vi "VCO-FM-1.vi"() -> ()   [LabVIEW 2012]
uses:
  <vilib>/Platform/TimedLoop/XDataNode/timing_clust.ctl
  <vilib>/Platform/TimedLoop/XDataNode/nitl_modes.ctl
  <vilib>/Platform/TimedLoop/XDataNode/wakeup.ctl
  <vilib>/rvi/FXPMathLib/basic elements/FxpIntAccumulator/subVIs/nifxpmath_IntAccumulator_SimConfig.ctl
  <vilib>/rvi/FXPMathLib/FxpSinAndCos/subVIs/nifxpmath_SinAndCos_SimConfig.ctl
  <vilib>/rvi/Emulation/niFpgaSctlEmulationRegisterWithScheduler.vi
  <vilib>/rvi/FXPMathLib/basic elements/FxpIntAccumulator/simVIs/DllFxpIntAccumulator_sub.vi
  <vilib>/rvi/Emulation/niFpgaSctlEmulationScheduler.vi
  <vilib>/rvi/interface/RandomDataEmulation/nirviRandomDataFPGAFIFO.vi
  <vilib>/rvi/interface/RandomDataEmulation/niFpgaRandomDataHandleErrors.vi
  <vilib>/rvi/eio/common/nirviEmuTemplateMethod_errors.vi
  <vilib>/rvi/FXPMathLib/FxpSinAndCos/simVIs/DllFxpSinAndCosTemp_sub.vi
  <vilib>/Platform/TimedLoop/XDataNode/XDataNode.xnode
  <vilib>/rvi/FXPMathLib/basic elements/FxpIntAccumulator/XNode/nifxpmath_IntAccumulator.xnode
  <vilib>/rvi/FXPMathLib/FxpMul/XNode/nifxpmath_Multiplier.xnode
  <vilib>/rvi/DataTransferAndStorage/Container/XNode/niFpgaContainer.xnode
  <vilib>/rvi/interface/RandomDataEmulation/nirviRandomDataFpgaReadWriteTemplate.vi
  <vilib>/eio/EIONode/EIONode.xnode
  <vilib>/rvi/FXPMathLib/FxpSinAndCos/XNode/nifxpmath_SinAndCos.xnode
  <vilib>/Platform/TimedLoop/XDataNode/XDNodeRunTimeDep.lvlib
  <vilib>/rvi/FXPMathLib/sim/FxpSim.dll
panel:
  out "Numeric 3":fxp<+/-,64,2>
  out "Numeric 2":fxp<+/-,64,14>
  out "Z Indicator":fxp<+/-,64,12>
  out "Numeric":fxp<+/-,64,12>
  in  "Z":fxp<+/-,64,11>
  out "Ticks":i16
  in  "DAQ Acquisition Rate":i16
  out "Test Input":fxp<+/-,64,32>
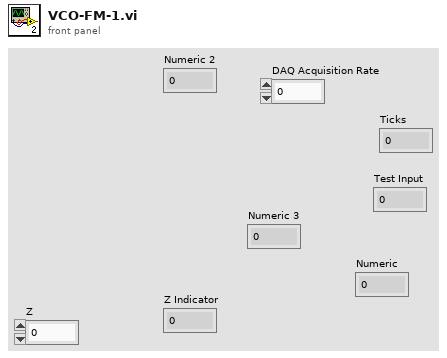
[diagram p1: front panel]
types:
  T1 = typedef "XDNodeRunTimeDep.lvlib/timing_clust.ctl" = cluster{"Expected End [f-1]":u64, "Actual End [f-1]":u64, "Finished Late? [f-1]":bool, "Expected End [i-1]":u64, "Actual End [i-1]":u64, "Finished Late? [i-1]":bool, "Expected Start [i]":u64, "Actual Start [i]":u64, "Expected Start [f]":u64, "Actual Start [f]":u64, "Source Name":string, "Structure Name":string, "Period":i64, "Deadline":i64, "Offset":i64, "Start":i64, "Priority":i32, "Timeout":i32, "Mode":T2, "Wakeup Reason":T3, "Error":errorcluster, "Source Type":string, "Secondary Source Type":string, "Global End Time":u64, "Global Start Time":u64, "Frame Duration":u64, "Iteration Duration":u64, "Assigned CPU":i32, "I/O Scan Engine Mode":u32}
  T2 = typedef "XDNodeRunTimeDep.lvlib/nitl_modes.ctl" = enum32{"No Change", "Process missed periods, maintain original phase", "Discard missed periods, maintain original phase", "Process missed periods, ignore original phase", "Discard missed periods, ignore original phase"}
  T3 = typedef "XDNodeRunTimeDep.lvlib/wakeup.ctl" = enum32{"Normal", "Aborted", "Asynchronous wakeup", "Timing source error", "Timed loop error", "Timeout"}
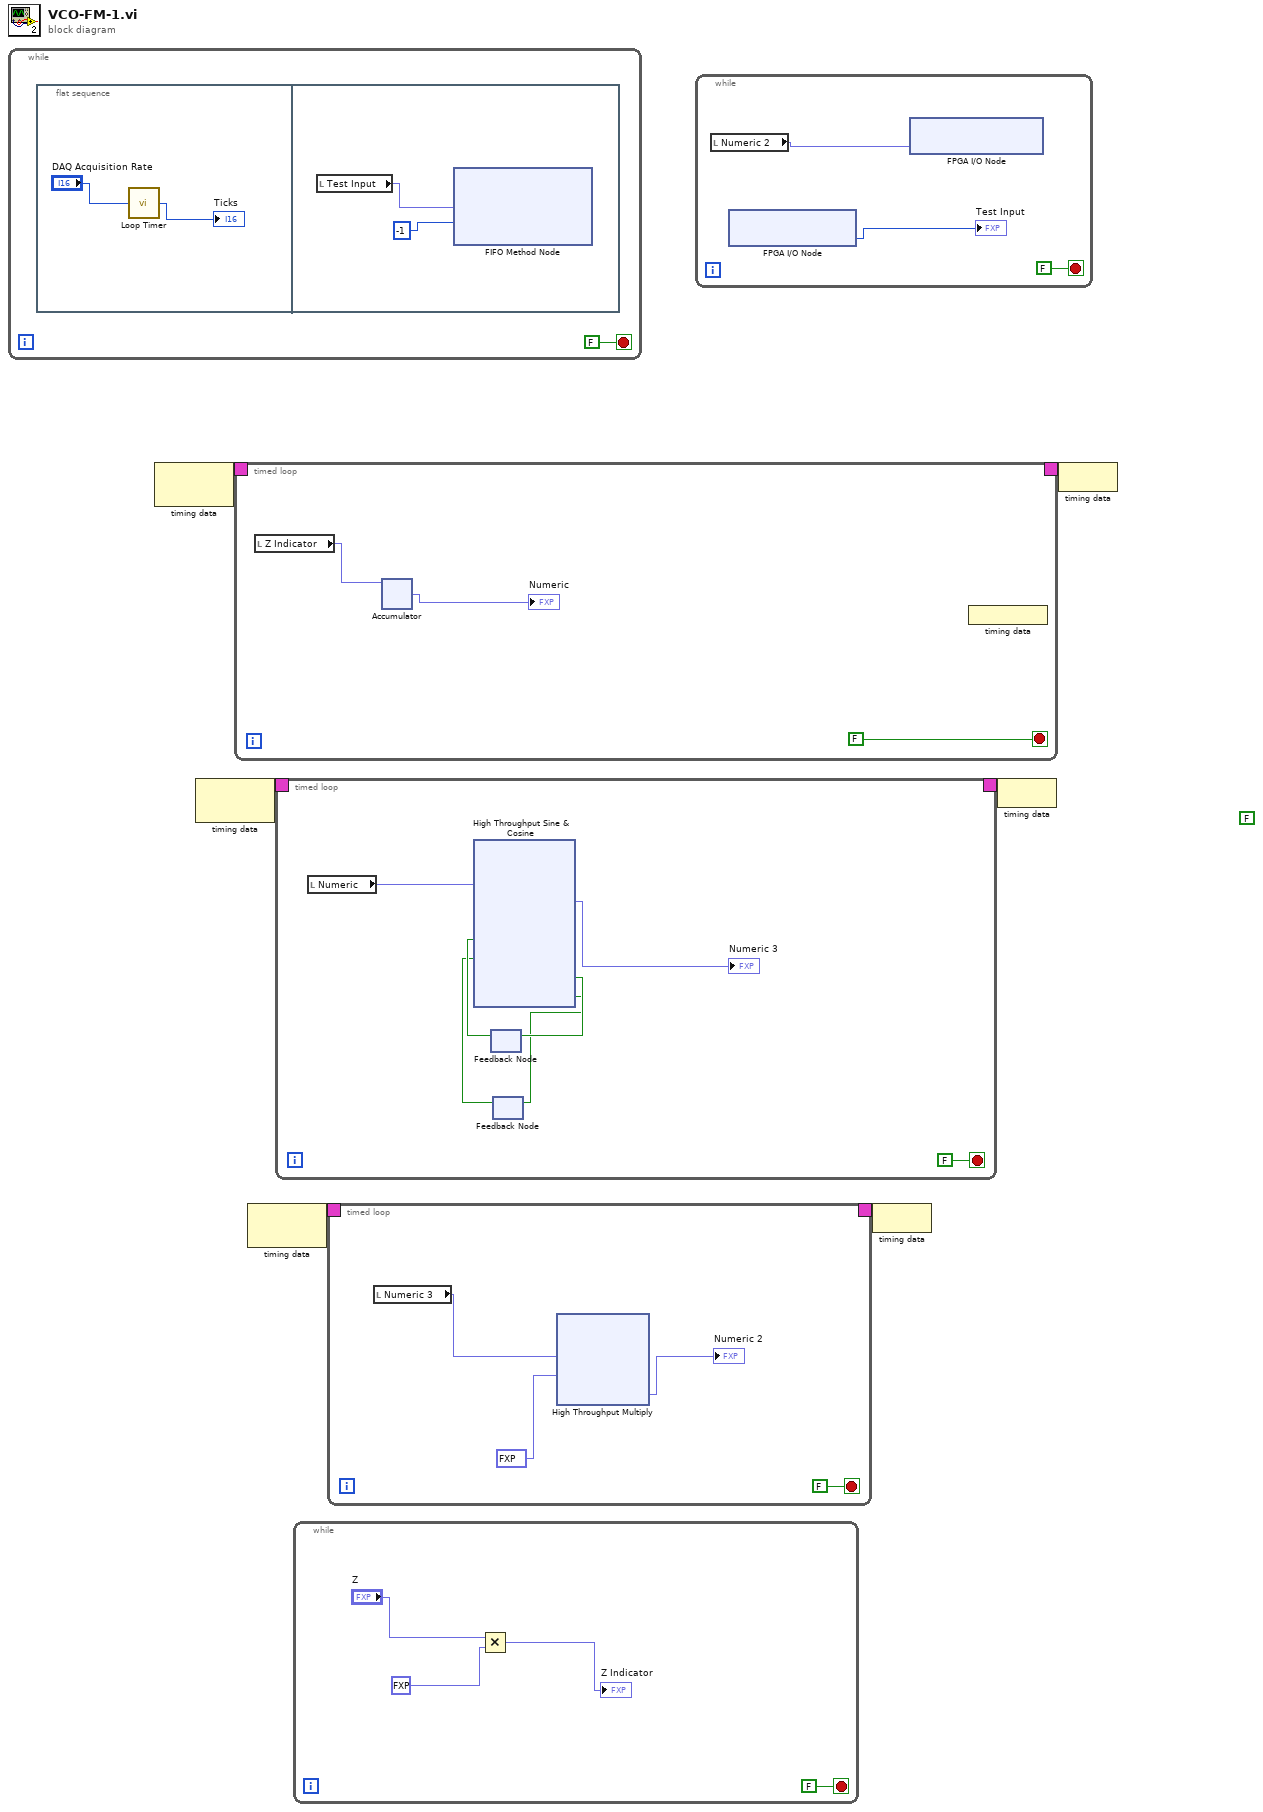
[diagram p0: block diagram]
diagram:
  (unwired) FALSE
  n1 = while {
    stop <- FALSE stop-if-true
    n2 = flat-sequence {
      frame #0 {
        n3 = call "Loop Timer"("Count(uSec)"="DAQ Acquisition Rate") -> ("Tick Count(uSec)"=→"Ticks":u32)
      }
      frame #1 {
        n4 = local read "Test Input"() -> (w11:fxp<+/-,64,32>)
        n5 = xnode ("FIFO Method Node")("Element"=w11, "Timeout"=-1) -> ()  [unwired: 1 in, 2 out]
      }
    }
  }
  n6 = node-c288() -> (w4:T1)  [unwired: 1 in]
  n7 = node-c288() -> (w2:T1)  [unwired: 1 in]
  n8 = timed-loop {
    timing: w4 -> [_]
    timing-out: [_] -> w3
    stop <- FALSE stop-if-true
    n9 = local read "Z Indicator"() -> (w13:fxp<+/-,64,12>)
    n10 = xnode "Accumulator"("x"=w13) -> ("s"=→"Numeric":fxp<+/-,64,12>)  [unwired: 4 in, 1 out]
    n11 = node-c288() -> ()  [unwired: 1 out]
  }
  n12 = node-c288() -> (w6:T1)  [unwired: 1 in]
  n13 = timed-loop {
    timing: w2 -> [_]
    timing-out: [_] -> w1
    stop <- FALSE stop-if-true
    n14 = local read "Numeric"() -> (w46:fxp<+/-,64,12>)
    n15 = feedback #1() -> (w49:bool)  [unwired: 1 in]
    n16 = feedback #2() -> (w47:bool)  [unwired: 1 in]
    n17 = xnode ("High Throughput Sine & Cosine")("x (pi)"=w46, "input valid"=w49, "ready for output (T)"=w47) -> ("sin(x)"=→"Numeric 3":fxp<+/-,64,2>, "output valid"=w50:bool, "ready for input"=w48:bool)  [unwired: 1 out]
    n18 = feedback-in #1(w50) -> ()
    n19 = feedback-in #2(w48) -> ()
  }
  n20 = while {
    stop <- FALSE stop-if-true
    n21 = Multiply(x="Z", y=fxp<+,1,1> 1.0) -> (x*y=→"Z Indicator":fxp<+/-,64,11>)
  }
  n22 = timed-loop {
    timing: w6 -> [_]
    timing-out: [_] -> w5
    stop <- FALSE stop-if-true
    n23 = local read "Numeric 3"() -> (w91:fxp<+/-,64,2>)
    n24 = xnode ("High Throughput Multiply")("x"=w91, "y"=fxp<+,10,12> 3276.0) -> ("x*y"=→"Numeric 2":fxp<+/-,64,14>)
  }
  n25 = while {
    stop <- FALSE stop-if-true
    n26 = local read "Numeric 2"() -> (w95:fxp<+/-,64,14>)
    n27 = xnode "FPGA I/O Node"() -> ("Connector0/AI6"=→"Test Input":i16)  [unwired: 1 in, 1 out]
    n28 = xnode "FPGA I/O Node"("Connector0/AO2"=w95) -> ()  [unwired: 1 in, 1 out]
  }
  n29 = node-c288(w5) -> ()
  n30 = node-c288(w1) -> ()
  n31 = node-c288(w3) -> ()
